vi "test_libssh2_session_last_errno.vi"() -> ()   [LabVIEW 2013, in "libssh2_integration_tests.lvlib"]
uses:
  libssh2_integration_tests.lvlib
  <vilib>/addons/_JKI Toolkits/Caraya/classes/Test/Test.lvclass
  <vilib>/addons/_JKI Toolkits/Caraya/classes/Assert/Assert.lvclass
  libssh2/libssh2.lvlib
panel:
  out "error out":errorcluster
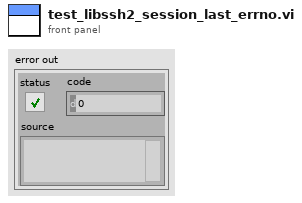
[diagram p1: front panel]
types:
  T1 = cluster{"error code":i32, "error message":string}[]
  T2 = typedef "libssh2.lvlib/Session Refnum.ctl" = refnum<k1>
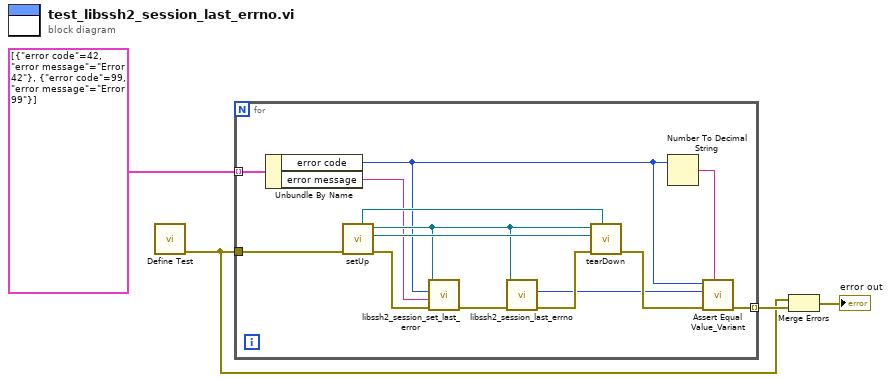
[diagram p0: block diagram]
diagram:
  n1 = call <vilib>:"Define Test.vi"() -> ("error out"=w2:errorcluster)  [unwired: 10 in, 1 out]
  n2 = for {
    tunnel: [w18] -> w4 mode=indexing
    tunnel: w2 -> [w17]
    tunnel: T1 [{"error code"=42, "error message"="Error 42"}, {"error code"=99, "error message"="Error 99"}] -> [w9] mode=indexing
    n3 = Unbundle By Name(w9) -> ("error code"=w6:i32, "error message"=w8:string)
    n4 = call "setUp.vi"("error in (no error)"=w17) -> ("error out"=w13:errorcluster, "connection ID"=w16:refnum<k5>, "session"=w10:T2, "fixture"=w15:refnum<class "Server Fixture.lvclass">)  [unwired: 7 in]
    n5 = call "libssh2_session_set_last_error.vi"("error in (no error)"=w13, "error message"=w8, "error code"=w6, "session"=w10) -> ("error out"=w14:errorcluster)  [unwired: 7 in]
    n6 = call "libssh2_session_last_errno.vi"("error in (no error)"=w14, "session"=w10) -> ("error out"=w11:errorcluster, "error code"=w7:i32)  [unwired: 8 in]
    n7 = call "tearDown.vi"("fixture"=w15, "error in (no error)"=w11, "connection ID"=w16, "session"=w10) -> ("error out"=w12:errorcluster)  [unwired: 7 in]
    n8 = Number To Decimal String(number=w6) -> (decimal integer string=w5:string)  [unwired: 1 in]
    n9 = call <vilib>:"Assert Equal Value_Variant.vi"("Label"=w5, "error in (no error)"=w12, "Y"=w7, "X"=w6) -> ("error out"=w18:errorcluster)  [unwired: 6 in, 1 out]
  }
  n10 = Merge Errors(w2, w4) -> (→"error out":errorcluster)
